vi "System_Initialize_Tags.vi"(11 "System DVR":refnum<data-value>) -> (2 "TagDescriptions":refnum<class "tag descriptor.lvclass">[](array[class]), 3 "System DVR out":refnum<data-value>)   [LabVIEW 2015, in "System.lvclass"]
uses:
  System.lvclass
  <vilib>/NI/Tag Bus/tag/tag descriptor.lvclass
  System.lvclass/System.ctl
  AssetInterface/Interface_Asset.lvclass
  DispatchInterface/Interface_Dispatch.lvclass
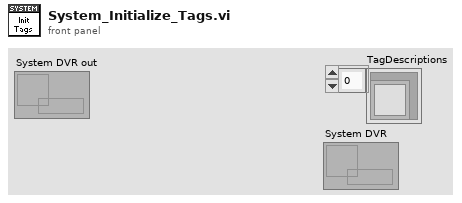
[diagram p1: front panel]
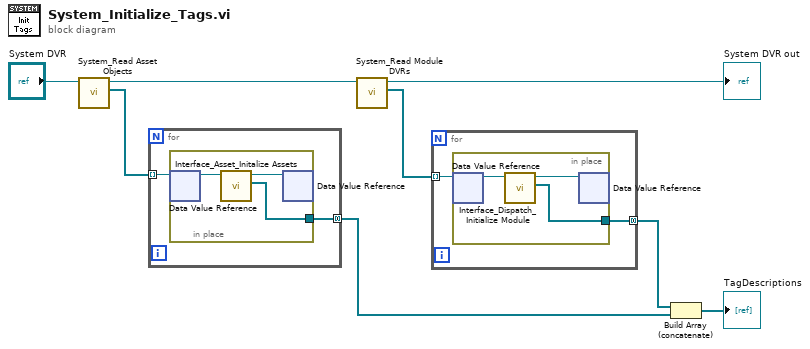
[diagram p0: block diagram]
diagram:
  n1 = call "System_Read Asset Objects.vi"("data value reference"="System DVR") -> ("Asset DVR Array"=w7:refnum<data-value>[], "data value reference out"=w4:refnum<data-value>)  [unwired: 9 in]
  n2 = for {
    tunnel: w7 -> [w10] mode=indexing
    tunnel: [w9] -> w6 mode=concatenating
    n3 = in-place {
      in-place-border: [w13] -> w9
      n4 = in-place-dvr #1(w10) -> (w12:refnum<class "Interface_Asset.lvclass">)  [unwired: 1 out]
      n5 = call-dynamic "Interface_Asset_Initalize Assets.vi"("AssetInterface in"=w12) -> ("TagDescriptions"=w13:refnum<class "tag descriptor.lvclass">[], "AssetInterface out"=w11:refnum<class "Interface_Asset.lvclass">)  [unwired: 8 in, 1 out]
      n6 = in-place-dvr #1(w11) -> ()  [unwired: 2 out]
    }
  }
  n7 = call "System_Read Module DVRs.vi"("Data Value Reference in"=w4) -> ("Dispatch Module DVR Array"=w1:refnum<data-value>[], "Data Value Reference out"=→"System DVR out":refnum<data-value>)  [unwired: 9 in]
  n8 = for {
    tunnel: w1 -> [w15] mode=indexing
    tunnel: [w14] -> w2 mode=concatenating
    n9 = in-place {
      in-place-border: [w17] -> w14
      n10 = in-place-dvr #2(w15) -> (w18:refnum<class "Interface_Dispatch.lvclass">)  [unwired: 1 out]
      n11 = call-dynamic "Interface_Dispatch_Initialize Module.vi"("Interface_Dispatch in"=w18) -> ("TagDescriptions"=w17:refnum<class "tag descriptor.lvclass">[], "Interface_Dispatch out"=w16:refnum<class "Interface_Dispatch.lvclass">)  [unwired: 8 in, 1 out]
      n12 = in-place-dvr #2(w16) -> ()  [unwired: 2 out]
    }
  }
  n13 = Build Array (concatenate)(w2, w6) -> (→"TagDescriptions":refnum<class "tag descriptor.lvclass">[])
